vi "test Deploy Scripted Custom Device with One Channel.vi"(8 "error in (no error)":errorcluster, 11 "TestCase in":refnum<class "Embedded Data Logger Scripting System Tests.lvclass">) -> (0 "error out":errorcluster, 3 "TestCase out":refnum<class "Embedded Data Logger Scripting System Tests.lvclass">)   [LabVIEW 2027, in "Embedded Data Logger Scripting System Tests.lvclass"]
uses:
  Embedded Data Logger Scripting System Tests.lvclass
  Embedded Data Logger Scripting System Tests.lvclass/Embedded Data Logger Scripting System Tests.ctl
  <vilib>/addons/_JKI Toolkits/VI Tester/TestCase.llb/TestCase.lvclass
  30dc589a-39cd-48ac-8e8d-4a58a160e88c.vi
  <vilib>/NI/VeriStand Custom Device Testing Tools/VeriStandTestUtilities/VeriStandTestUtilities.lvlib
  Embedded Data Logger Scripting.lvlib
  C:/NetCoreDLL/NationalInstruments.VeriStand.SystemDefinitionAPI.dll
  NetCoreDLL/NationalInstruments.VeriStand.SystemDefinitionAPI.dll
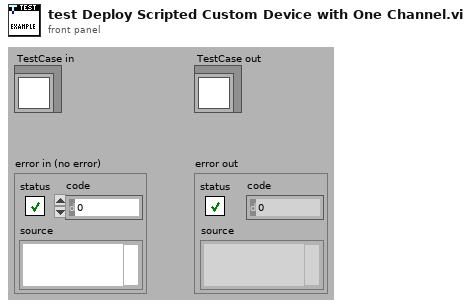
[diagram p1: front panel]
types:
  T1 = typedef "Custom Device API.lvlib/Custom Device Item Ref.ctl" = u64
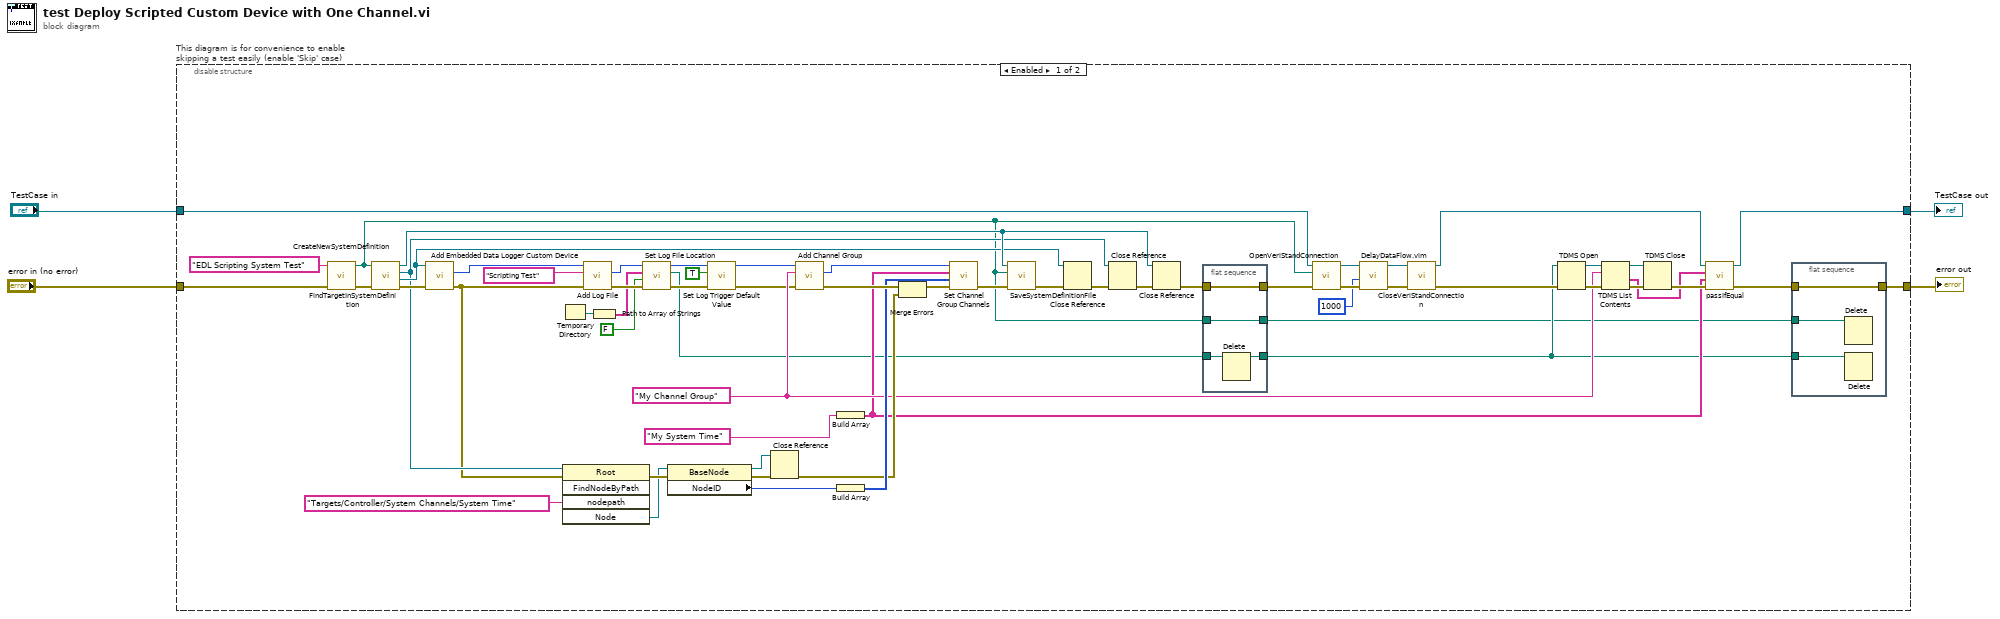
[diagram p0: block diagram]
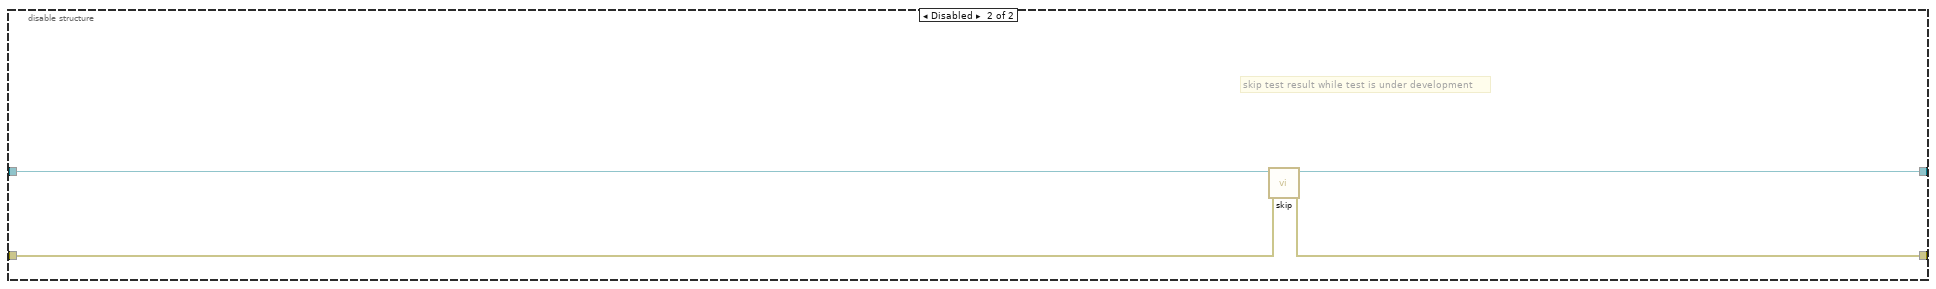
[diagram p2: hidden frame]
diagram:
  n1 = disable-structure "This diagram is for convenience to enable skipping a test easily (enable 'Skip' case)" shown="Enabled" {
    disable-tunnel: "TestCase in" -> [w64 w75]
    disable-tunnel: [w15 w73] -> w1
    disable-tunnel: [w50 w74] -> w3
    disable-tunnel: "error in (no error)" -> [w59 w72]
    frame Enabled {
      w18 = "My Channel Group" ("group name")
      n2 = call <vilib>:"CreateNewSystemDefinition.vi"("error in"=w59, "System Definition Name"="EDL Scripting System Test") -> ("error out"=w58:errorcluster, "System Definition Path"=w8:path)  [unwired: 8 in]
      n3 = call <vilib>:"FindTargetInSystemDefinition.vi"("error in"=w58, "system definition path"=w8) -> ("error out"=w55:errorcluster, "NationalInstruments.VeriStand.SystemDefinitionAPI.Target"=w37:refnum<k39>, "NationalInstruments.VeriStand.SystemDefinitionAPI.Root"=w28:refnum<k39>, "NationalInstruments.VeriStand.SystemDefinitionAPI.SystemDefinition"=w38:refnum<k39>)  [unwired: 6 in]
      n4 = call "Add Embedded Data Logger Custom Device.vi"("error in"=w55, "NationalInstruments.VeriStand.SystemDefinitionAPI.Target"=w37) -> ("error out"=w22:errorcluster, "embedded data logger"=w44:T1)  [unwired: 7 in, 1 out]
      n5 = Temporary Directory() -> (w51:path)
      n6 = invoke class="Root" method="FindNodeByPath"(reference=w28, error in=w22, "nodepath"="Targets/Controller/System Channels/System Time" ("Item Path in")) -> (error out=w27:errorcluster, "Node"=w26:refnum<k39>)  [unwired: 2 in, 3 out]
      n7 = call "Add Log File.vi"("error in"=w22, "log file name"="Scripting Test", "embedded data logger in"=w44) -> ("error out"=w54:errorcluster, "log file"=w20:T1)  [unwired: 6 in, 1 out]
      n8 = Path to Array of Strings(0:w51) -> (2:w53:string[])  [unwired: 1 out]
      n9 = call "Set Log File Location.vi"("error in"=w54, "timestamp file name"=FALSE, "directory parts"=w53, "log file in"=w20) -> ("error out"=w49:errorcluster, "sample path"=w12:path, "log file out"=w48:T1)  [unwired: 5 in]
      n10 = property class="BaseNode"(reference=w26, error in=w27) -> (reference out=w25:refnum<k39>, error out=w24:errorcluster, "NodeID"=w23:u64)
      n11 = call "Set Log Trigger Default Value.vi"("error in"=w49, "log trigger default value"=TRUE, "log file in"=w48) -> ("error out"=w5:errorcluster, "log file out"=w6:T1)  [unwired: 7 in]
      n12 = Close Reference(reference=w25, error in (no error)=w24) -> (error out=w21:errorcluster)
      n13 = call "Add Channel Group.vi"("error in"=w5, "group name"=w18, "log file in"=w6) -> ("error out"=w46:errorcluster, "channel group"=w19:T1)  [unwired: 6 in, 1 out]
      n14 = Build Array("My System Time" ("Item Path in")) -> (w13:string[])
      n15 = Build Array(w23) -> (w42:u64[])
      n16 = Merge Errors(w46, w21) -> (w43:errorcluster)
      n17 = call "Set Channel Group Channels.vi"("error in"=w43, "channels"=w42, "names"=w13, "channel group in"=w19) -> ("error out"=w45:errorcluster)  [unwired: 4 in, 3 out]
      n18 = call <vilib>:"SaveSystemDefinitionFile.vi"("error in (no error)"=w45, "System Definition File in"=w8, "NationalInstruments.VeriStand.SystemDefinitionAPI.SystemDefinition"=w38) -> ("error out"=w56:errorcluster)  [unwired: 7 in, 1 out]
      n19 = Close Reference(reference=w37, error in (no error)=w56) -> (error out=w39:errorcluster)
      n20 = Close Reference(reference=w28, error in (no error)=w39) -> (error out=w40:errorcluster)
      n21 = Close Reference(reference=w38, error in (no error)=w40) -> (error out=w9:errorcluster)
      n22 = flat-sequence {
        tunnel: w12 -> [w68]
        tunnel: [w67] -> w11
        tunnel: [w66] -> w10
        tunnel: w9 -> [w66]
        tunnel: w8 -> [w65]
        tunnel: [w65] -> w7
        frame #0 {
          n23 = Delete(path (use dialog)=w68) -> (deleted path=w67:path)  [unwired: 4 in, 2 out]
        }
      }
      n24 = call-dynamic "OpenVeriStandConnection.vi"("error in (no error)"=w10, "System Definition File"=w8, "VeriStand Test Case in"=w64) -> ("error out"=w62:errorcluster, "VeriStand Test Case out"=w63:refnum<class "Embedded Data Logger Scripting System Tests.lvclass">)  [unwired: 6 in, 1 out]
      n25 = call "DelayDataFlow.vim"("value in"=w62, "milliseconds to wait"=u32 1000) -> ("value out"=w61:errorcluster)  [unwired: 2 in, 1 out]
      n26 = call-dynamic "CloseVeriStandConnection.vi"("error in (no error)"=w61, "VeriStand Test Case in"=w63) -> ("error out"=w41:errorcluster, "VeriStand Test Case out"=w16:refnum<class "Embedded Data Logger Scripting System Tests.lvclass">)  [unwired: 8 in]
      n27 = TDMS Open(8:w41, 11:w11) -> (0:w35:errorcluster, 3:w32:refnum<k34>)  [unwired: 5 in]
      n28 = TDMS List Contents(4:w35, 6:w18, 7:w32) -> (0:w33:errorcluster, 1:w14:string[], 3:w30:refnum<k34>)  [unwired: 1 out]
      n29 = TDMS Close(8:w33, 11:w30) -> (0:w31:errorcluster)  [unwired: 1 out]
      n30 = call-dynamic "passIfEqual.vi"("error in (no error)"=w31, "y"=w13, "x"=w14, "TestCase in"=w16) -> ("error out"=w17:errorcluster, "TestCase out"=w15:refnum<class "Embedded Data Logger Scripting System Tests.lvclass">)  [unwired: 6 in]
      n31 = flat-sequence {
        tunnel: w7 -> [w69]
        tunnel: w11 -> [w71]
        tunnel: [w70] -> w50
        tunnel: w17 -> [w70]
        frame #0 {
          n32 = Delete(path (use dialog)=w69) -> ()  [unwired: 4 in, 3 out]
          n33 = Delete(path (use dialog)=w71) -> ()  [unwired: 4 in, 3 out]
        }
      }
    }
    frame Disabled {
      # "skip test result while test is under development"
      n34 = call <vilib>:"skip.vi"("error in (no error)"=w72, "TestCase in"=w75) -> ("error out"=w74:errorcluster, "TestCase out"=w73:refnum<class "Embedded Data Logger Scripting System Tests.lvclass">)  [unwired: 8 in]
    }
  }
  "error out" <- w3
  "TestCase out" <- w1
